vi "PWM.Generate.Digital.Convert.vi"(11 "Settings":T1={"ACTIVE EDGE"=TRUE, "FREQ"=0.0, "DC"=0.0}) -> (3 "Settings":T2)   [LabVIEW 2019, in "Speciality FPGA IO.lvlib"]
uses:
  Speciality FPGA IO.lvlib
  Types/PWM.Generate.Digital.Settings.ctl
  Types/PWM.Generate.Digital.Convert.Settings.ctl
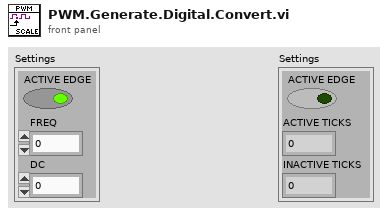
[diagram p1: front panel]
types:
  T1 = typedef "Speciality FPGA IO.lvlib/PWM.Generate.Digital.Convert.Settings.ctl" = cluster{"ACTIVE EDGE":bool, "FREQ":sgl, "DC":sgl}
  T2 = typedef "Speciality FPGA IO.lvlib/PWM.Generate.Digital.Settings.ctl" = cluster{"ACTIVE EDGE":bool, "ACTIVE TICKS":u32, "INACTIVE TICKS":u32}
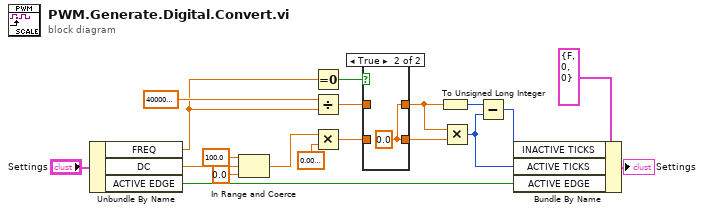
[diagram p0: block diagram]
diagram:
  n1 = Unbundle By Name("Settings") -> ("FREQ"=w10:sgl, "DC"=w3:sgl, "ACTIVE EDGE"=w11:bool)
  n2 = In Range and Coerce(upper limit=sgl 100.0, x=w3, lower limit=sgl 0.0) -> (coerced(x)=w4:sgl)  [unwired: 1 out]
  n3 = Equal To 0?(x=w10) -> (x = 0?=w9:bool)
  n4 = Divide(x=sgl 40000000.0 ("y"), y=w10) -> (x/y=w8:sgl)
  n5 = Multiply(x=w4, y=sgl 0.01 ("x")) -> (x*y=w5:sgl)
  n6 = case shown="True" w9 {
    tunnel: w8 -> [w21 _]
    tunnel: [w21 w22] -> w7
    tunnel: [w20 w22] -> w6
    tunnel: w5 -> [w20 _]
    frame False {
    }
    frame True {
      w22 = sgl 0.0
    }
  }
  n7 = To Unsigned Long Integer(number=w7) -> (unsigned 32bit integer=w18:u32)
  n8 = Multiply(x=w7, y=w6) -> (x*y=w14:u32)
  n9 = Subtract(x=w18, y=w14) -> (x-y=w15:u32)
  n10 = Bundle By Name(cluster=T2 {"ACTIVE EDGE"=FALSE, "ACTIVE TICKS"=0, "INACTIVE TICKS"=0} ("Channel.Settings"), "INACTIVE TICKS"=w15, "ACTIVE TICKS"=w14, "ACTIVE EDGE"=w11) -> (→"Settings":T2)
